vi "get Julia ZMQ server path.vi"(8 "error in (no error)":errorcluster, 11 "Julia ZMQ server file name":string="ZMQ-testserver2.jl") -> (0 "error out":errorcluster, 3 "Julia ZMQ server file path":path)   [LabVIEW 2018, in "LV-Julia_ZMQ-Roundtrip_lib.lvlib"]
uses:
  LV-Julia_ZMQ-Roundtrip_lib.lvlib
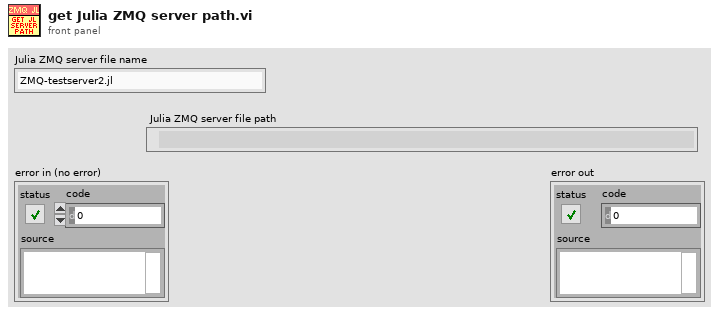
[diagram p1: front panel]
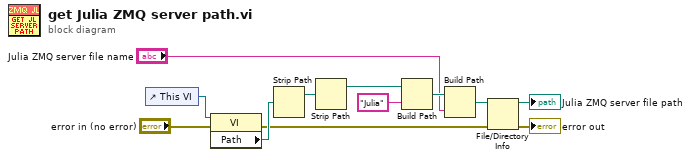
[diagram p0: block diagram]
diagram:
  n1 = control-ref of="This VI"() -> (w12:refnum<vi>)
  n2 = property class="VI"(reference=w12, error in="error in (no error)") -> (error out=w3:errorcluster, "Path"=w10:path)  [unwired: 1 out]
  n3 = Strip Path(path=w10) -> (stripped path=w9:path)  [unwired: 1 out]
  n4 = Strip Path(path=w9) -> (stripped path=w8:path)  [unwired: 1 out]
  n5 = Build Path(base path=w8, name or relative path="Julia") -> (appended path=w7:path)
  n6 = Build Path(base path=w7, name or relative path="Julia ZMQ server file name") -> (appended path=w4:path)
  n7 = File/Directory Info(path=w4, error in=w3) -> (path out=→"Julia ZMQ server file path":path, error out=→"error out":errorcluster)  [unwired: 5 out]
